vi "HLP_Query.vi"(0 "System no.":i32=1 min=1 max=4 step=1, 5 "error in":errorcluster) -> (14 "Help string":string, 19 "error out":errorcluster)   [LabVIEW 2020]
doc: "GCS 3.0\n=====\n\nHLP? (Get List Of Available Commands)\n\nDescription\nLists all commands supported by the controller.\n\nFormat\nHLP?\n\nArguments\nnone\n\nResponse\nA list of all commands that can be executed in the current user command level. The list has the \nfollowing format:\nThe following commands are valid:\nCommand Arguments Description LF\n...\nend of help\nThe second to penultimate lines of the list each describe a command using the following \ncomponents:\n- Command Command mnemonic\n- Arguments Syntax for the arguments of the command. The value \"-\" means that the \ncommand does not have any arguments.\n- Description Description of the command\n\nExample\n>>HLP?\n<<The following commands are valid:\n<<CPA <SourceMemoryType> <DestinationMemoryType> [<Container\nUnit> [<Function Unit> [<ParameterID>]]] Copy value of\nspecified ParameterID from Memory Source to Memory Destination\n<<CSV? - Get GCS Version\n[...]\n<<VER? - Get Versions of Firmware, UMF and Drivers\n<<XXX - Timing CMD (PI internal only)\n<<end of help\n\nNotes\nDetailed descriptions of the commands and keywords for section commands must be queried \nwith the USG? CMD command. \nFrom the second to penultimate line, the response to HLP? is identical to the Command \nOverview block in the response to the USG? CMD command, if this command is sent without \narguments.\n\nUser command level\nUSR\n\n\nGCS 2.0\n=====\n\nReturns help string. \n\nC-887, F-206, M-8X0: For GCS syntax version = GCS 1.0 (Check with CSV?.vi. If CSV?.vi is not supported, syntax version is GCS 1.0), check HELP answer to determine if HLP? is supported. HLP? and HELP are equivalent."
panel:
  # "HLP? (Get List Of Available Commands)\n\nLists all commands supported by the controller."
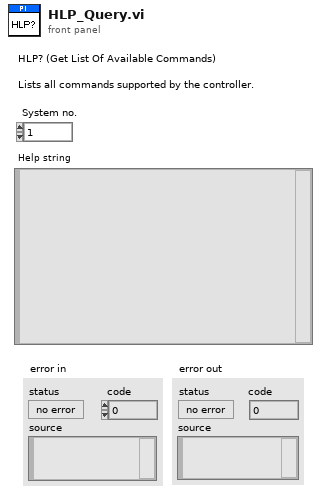
[diagram p1: front panel]
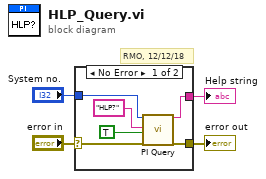
[diagram p0: block diagram]
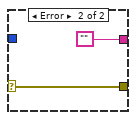
[diagram p2: hidden frame]
diagram:
  # "RMO, 12/12/18"
  n1 = case shown="No Error" "error in" {
    selector: "error in" -> [w7 w12]
    tunnel: [w5 ""] -> w4
    tunnel: [w6 w12] -> w3
    tunnel: "System no." -> [w8 _]
    frame No Error {
      n2 = call "PI Query.vi"("System no."=w8, "String to send"="HLP?" ("String to Send"), "Attach termination char.?"=TRUE ("Attach Linefeed?"), "error in"=w7) -> ("String read"=w5:string, "error out"=w6:errorcluster)  [unwired: 3 in, 11 out]
    }
    frame Error {
    }
  }
  "Help string" <- w4
  "error out" <- w3
